vi "SCCT Read X Orientation.vi"(0 "Publisher In":refnum<class "Publisher.lvclass">, 5 "timeout in ms(0)":i32=100, 11 "input cluster":errorcluster) -> (4 "Publisher Out":refnum<class "Publisher.lvclass">, 6 "X Orientation":dbl, 10 "XMLDocument":string, 13 "status":bool, 15 "error out 2":errorcluster)   [LabVIEW 2011]
uses:
  <vilib>/TOOLS FOR SMART MINDS/SCCT/Publisher/Publisher.lvclass
  <vilib>/TOOLS FOR SMART MINDS/SCCT/Publisher/Read XMLData.vi
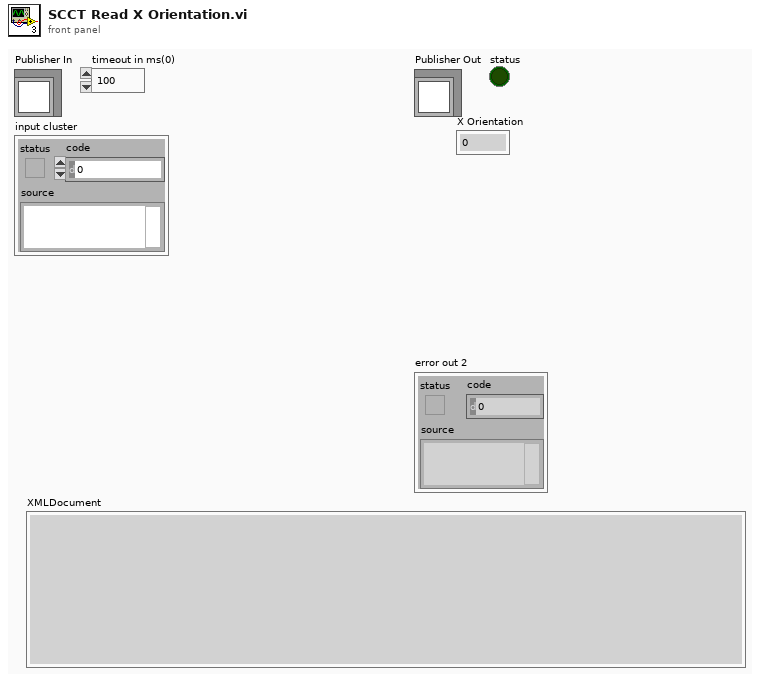
[diagram p1: front panel]
types:
  T1 = cluster{"timeStamp":timestamp, "value":cluster{"XMLDocument":string}, "senderAddress":string}
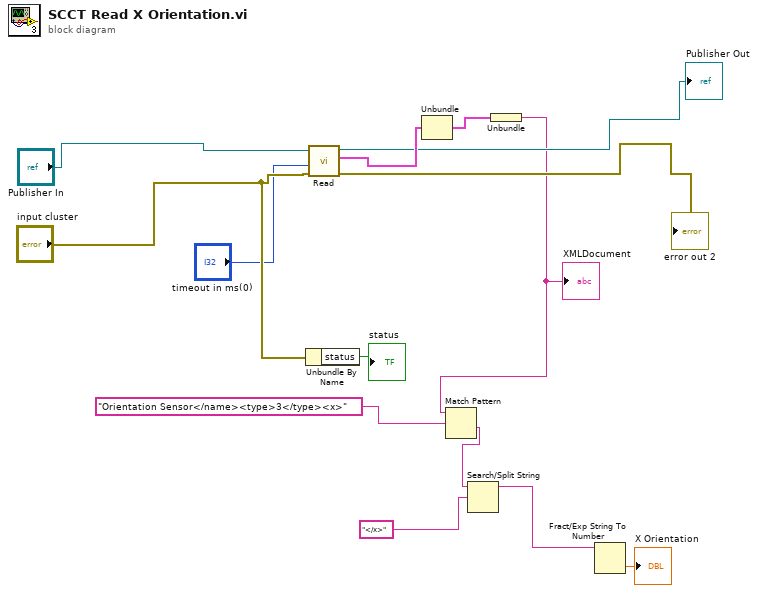
[diagram p0: block diagram]
diagram:
  n1 = Unbundle By Name("input cluster") -> ("status"=→"status":bool)
  n2 = call-poly <vilib>:"Read.vi"("error in (no error)"="input cluster", "timeout in ms(0)"="timeout in ms(0)", "Publisher In"="Publisher In") -> ("error out"=→"error out 2":errorcluster, "customXMLData"=w14:T1, "Publisher Out"=→"Publisher Out":refnum<class "Publisher.lvclass">)  [unwired: 4 in, 2 out]
  n3 = Unbundle(w14) -> ("value"=w13:cluster{"XMLDocument":string})  [unwired: 2 out]
  n4 = Unbundle(w13) -> ("XMLDocument"=w3:string)
  "XMLDocument" <- w3
  n5 = Match Pattern(string=w3, regular expression="Orientation Sensor</name><type>3</type><x>") -> (after substring=w10:string)  [unwired: 1 in, 3 out]
  n6 = Search/Split String(string=w10, search string/char (-)="</x>") -> (substring before match=w2:string)  [unwired: 1 in, 2 out]
  n7 = Fract/Exp String To Number(string=w2) -> (number=→"X Orientation":dbl)  [unwired: 3 in, 1 out]
